vi "Read XML_002.vi"(8 "error in (no error)":errorcluster, 10 "XML Configuration File Path":path=path "E:/Ballard - Arinc-429 CD/Example Database/Ballard/XML_000.XML") -> (0 "error IO":errorcluster, 3 "channels":T1 {"speed" items=["Auto", "Low", "High"]; "Labels"."scheduleBuildUnit" items=["Millisecond", "Microsecond"]})   [LabVIEW 2017, in "Ballard Arinc-429 System Explorer.lvlib"]
uses:
  Controls/Ballard_Channel Array.ctl
  Controls/Ballard_Channel.ctl
  Controls/Ballard_Label.ctl
  Controls/Ballard_Word.ctl
  Controls/ARINCParam.ctl
  Shared/Controls and Global/TransferType.ctl
  Controls/Channel_direction.ctl
  Controls/Channel Speed.ctl
  D:/Ballard-Arinc-429-Custom-Device/Source/System Explorer/SubVIs/Parse XML Ballard/Ballard_BTI_XML_Deserializer.dll
  Ballard_BTI_XML_Deserializer.dll
  Ballard Arinc-429 System Explorer.lvlib
  Shared/Ballard Arinc-429 Shared.lvlib
panel:
  out "name":string
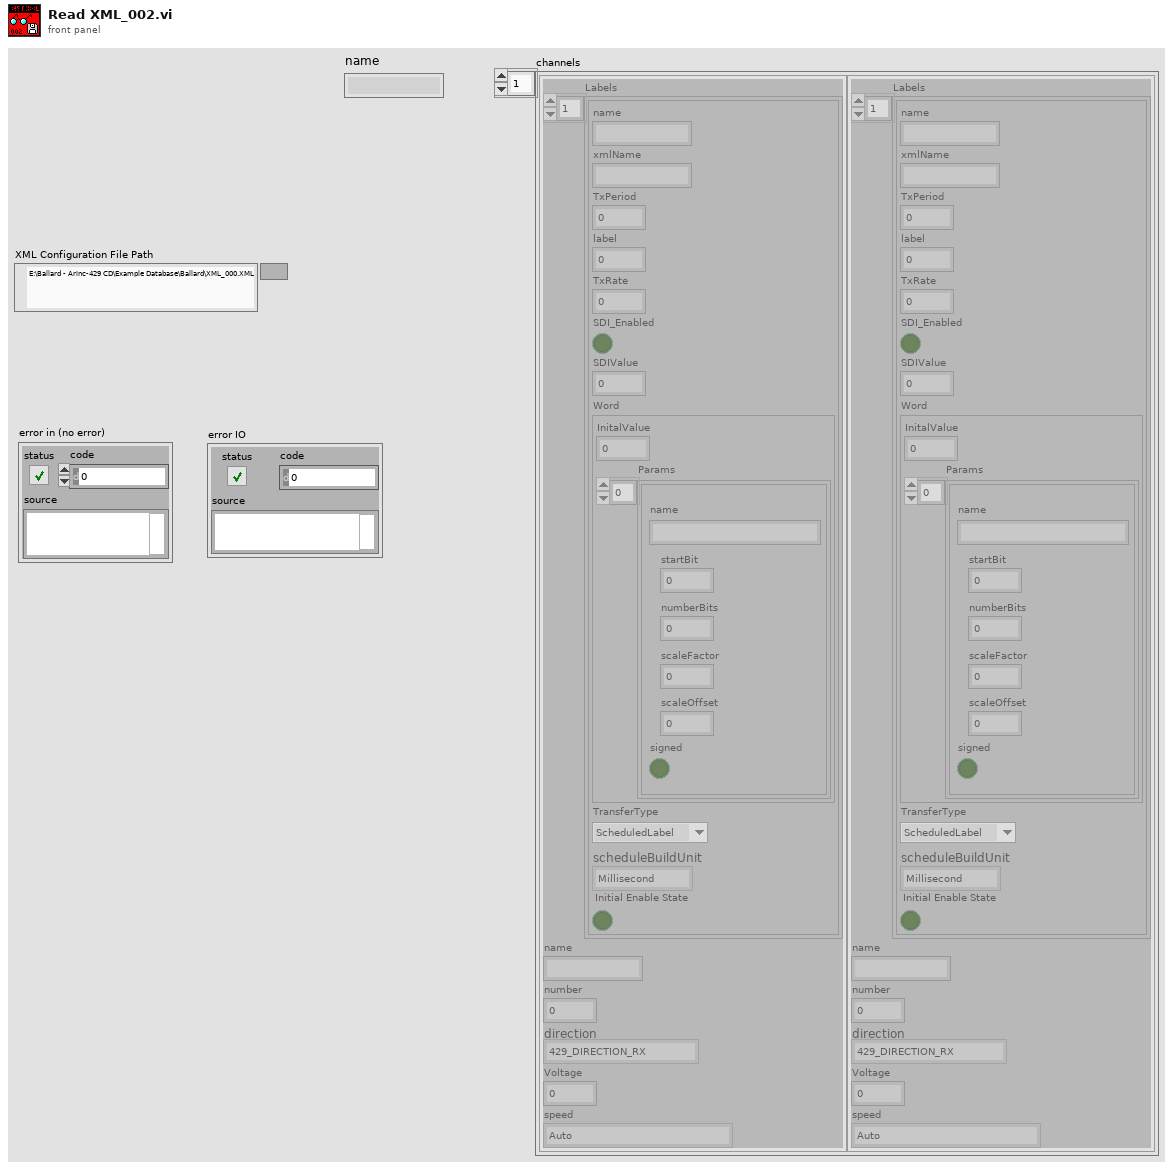
[diagram p1: front panel]
types:
  T1 = typedef "Ballard Arinc-429 System Explorer.lvlib/Ballard_Channel Array.ctl" = T2[]
  T2 = typedef "Ballard Arinc-429 System Explorer.lvlib/Ballard_Channel.ctl" = cluster{"Labels":T3[], "name":string, "number":u8, "direction":T7, "Voltage":dbl, "speed":T8}
  T3 = typedef "Ballard Arinc-429 System Explorer.lvlib/Ballard_Label.ctl" = cluster{"name":string, "xmlName":string, "TxPeriod":u32, "label":u32, "TxRate":dbl, "SDI_Enabled":bool, "SDIValue":u8, "Word":T4, "TransferType":T6, "scheduleBuildUnit":i32, "Initial Enable State":bool}
  T4 = typedef "Ballard Arinc-429 System Explorer.lvlib/Ballard_Word.ctl" = cluster{"InitalValue":u32, "Params":T5[]}
  T5 = typedef "Ballard Arinc-429 System Explorer.lvlib/ARINCParam.ctl" = cluster{"name":string, "startBit":i32, "numberBits":i32, "scaleFactor":dbl, "scaleOffset":dbl, "signed":bool}
  T6 = typedef "Ballard Arinc-429 Shared.lvlib/TransferType.ctl" = enum16{"ScheduledLabel", "Acyclic", "Block", "Strobe"}
  T7 = typedef "Ballard Arinc-429 System Explorer.lvlib/Channel_direction.ctl" = enum16{"429_DIRECTION_RX", "429_DIRECTION_TX"}
  T8 = typedef "Ballard Arinc-429 System Explorer.lvlib/Channel Speed.ctl" = i32
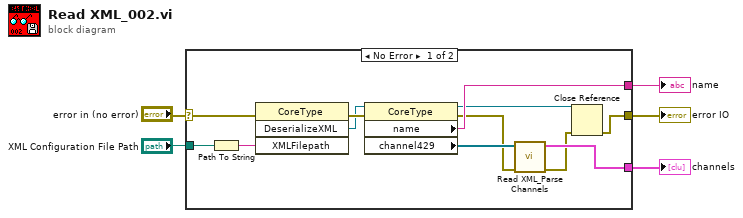
[diagram p0: block diagram]
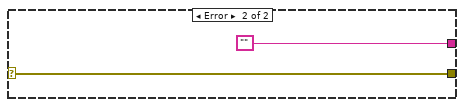
[diagram p2: hidden frame]
diagram:
  n1 = case shown="No Error" "error in (no error)" {
    selector: "error in (no error)" -> [w7 w19]
    tunnel: "XML Configuration File Path" -> [w17 _]
    tunnel: [w6 w19] -> w3
    tunnel: [w16 _] -> w2
    tunnel: [w15 "" ("name")] -> w1
    frame No Error {
      n2 = Path To String(path=w17) -> (string=w14:string)
      n3 = invoke class="CoreType" method="DeserializeXML"(error in=w7, "XMLFilepath"=w14) -> (error out=w9:errorcluster, "DeserializeXML"=w8:refnum<k24>)  [unwired: 2 in, 2 out]
      n4 = property class="CoreType"(reference=w8, error in=w9) -> (reference out=w10:refnum<k24>, error out=w12:errorcluster, "name"=w15:string, "channel429"=w13:refnum<k24>[])
      n5 = call "Read XML_Parse Channels.vi"("error in (no error)"=w12, "channel429"=w13) -> ("error out"=w11:errorcluster, "Array"=w16:T2[])  [unwired: 8 in]
      n6 = Close Reference(reference=w10, error in (no error)=w11) -> (error out=w6:errorcluster)
    }
    frame Error {
    }
  }
  "channels" <- w2
  "error IO" <- w3
  "name" <- w1
